vi "Teleop Drivetrain Control.vi"(10 "Button Cluster":T1, 11 "Axes":T2) -> ()   [LabVIEW 2015]
uses:
  Common Code/Gamepads/Axes Cluster.ctl
  Common Code/Gamepads/Button Cluster.ctl
  Common Code/Drivetrain Modes.ctl
  Common Code/Shot Type.ctl
  Common Code/Change Detect.vi
  Common Code/Change Detect Boolean.vi
  Robot Global Data.vi
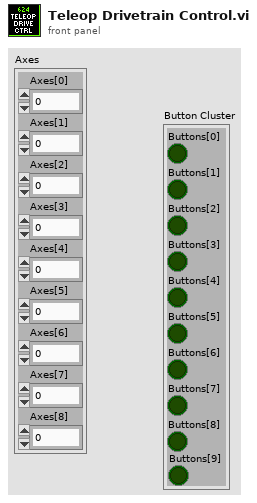
[diagram p1: front panel]
types:
  T1 = typedef "Button Cluster.ctl" = cluster{"Buttons[0]":bool, "Buttons[1]":bool, "Buttons[2]":bool, "Buttons[3]":bool, "Buttons[4]":bool, "Buttons[5]":bool, "Buttons[6]":bool, "Buttons[7]":bool, "Buttons[8]":bool, "Buttons[9]":bool}
  T2 = typedef "Axes Cluster.ctl" = cluster{"Axes[0]":dbl, "Axes[1]":dbl, "Axes[2]":dbl, "Axes[3]":dbl, "Axes[4]":dbl, "Axes[5]":dbl, "Axes[6]":dbl, "Axes[7]":dbl, "Axes[8]":dbl}
  T3 = typedef "Drivetrain Modes.ctl" = enum16{"Climb", "Manual", "Ball Vision Targeting", "Goal Vision Targeting", "PID Distance Drive", "Hybrid"}
  T4 = typedef "Shot Type.ctl" = enum16{"Batter Shot", "Corner Shot", "Curve Shot", "Vision Shot", "Deep Middle Shot"}
  T5 = typedef "Climb Command Cluster.ctl" = cluster{"Climb Mode":T6, "Hold?":bool, "Manual State":T7}
  T6 = typedef "Climb Mode.ctl" = enum16{"Auto", "Manual"}
  T7 = typedef "Climb Manual State.ctl" = cluster{"Release":bool, " PTO Engage":bool}
  T8 = typedef "Drivetrain Commands.ctl" = cluster{"Y Power":dbl, "Turn Power":dbl, "1st Gear?":bool, "Modes":T3, "Heading Target":dbl, "X Max Speed":dbl, "Y Max Speed":dbl, "X Min Speed":dbl, "Y Min Speed":dbl, "Y Target":dbl, "Max Accel":dbl, "Max Velocity":dbl}
  T9 = typedef "Shooter Command Cluster.ctl" = cluster{"Command":T10, "Mode":T11, "Shot Type":T4, "Override Trigger IR":bool}
  T10 = typedef "Shooter Commands.ctl" = enum16{"Idle", "Prime Shooter", "Shoot"}
  T11 = typedef "Shoot Modes Enum.ctl" = enum16{"Manual", "Safe", "Auto"}
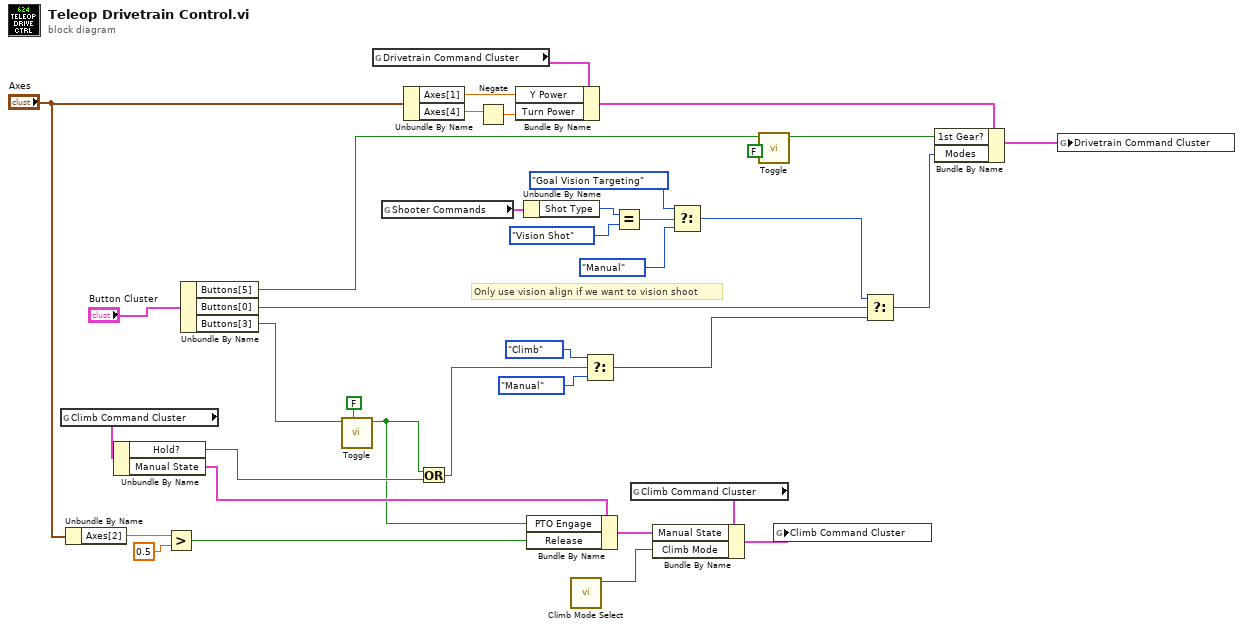
[diagram p0: block diagram]
diagram:
  # "Only use vision align if we want to vision shoot"
  n1 = global read "Robot Global Data.vi" "Climb Command Cluster"() -> (w17:T5)
  n2 = Unbundle By Name("Axes") -> ("Axes[2]"=w8:dbl)
  n3 = Unbundle By Name(w17) -> ("Hold?"=w16:bool, "Manual State"=w14:T7)
  n4 = Greater?(x=w8, y=0.5) -> (0:w6:bool)
  n5 = Unbundle By Name("Button Cluster") -> ("Buttons[5]"=w36:bool, "Buttons[0]"=w30:bool, "Buttons[3]"=w11:bool)
  n6 = call "Toggle.vi"("Initial Value"=FALSE, "In"=w11) -> ("Toggled"=w13:bool)  [unwired: 9 in]
  n7 = global read "Robot Global Data.vi" "Drivetrain Command Cluster"() -> (w31:T8)
  n8 = global read "Robot Global Data.vi" "Shooter Commands"() -> (w28:T9)
  n9 = Unbundle By Name("Axes") -> ("Axes[1]"=w4:dbl, "Axes[4]"=w3:dbl)
  n10 = Or(x=w13, y=w16) -> (x .or. y?=w15:bool)
  n11 = Negate(x=w3) -> (-x=w2:dbl)
  n12 = Bundle By Name(cluster=w31, "Y Power"=w4, "Turn Power"=w2) -> (w34:T8)
  n13 = Unbundle By Name(w28) -> ("Shot Type"=w27:T4)
  n14 = Bundle By Name(cluster=w14, "PTO Engage"=w13, "Release"=w6) -> (w12:T7)
  n15 = call "Climb Mode Select.vi"() -> ("Mode"=w5:T6)  [unwired: 11 in]
  n16 = Select(t=Drivetrain_Modes."Climb", s=w15, f=Drivetrain_Modes."Manual" ("Modes")) -> (s? t:f=w1:T3)
  n17 = Equal?(x=w27, y=Shot_Type."Vision Shot") -> (x = y?=w25:bool)
  n18 = global read "Robot Global Data.vi" "Climb Command Cluster"() -> (w18:T5)
  n19 = Bundle By Name(cluster=w18, "Manual State"=w12, "Climb Mode"=w5) -> (w10:T5)
  n20 = Select(t=Drivetrain_Modes."Goal Vision Targeting" ("Modes"), s=w25, f=Drivetrain_Modes."Manual") -> (s? t:f=w22:T3)
  n21 = call "Toggle.vi"("Initial Value"=FALSE, "In"=w36) -> ("Toggled"=w33:bool)  [unwired: 9 in]
  n22 = global write "Robot Global Data.vi" "Climb Command Cluster"(w10) -> ()
  n23 = Select(t=w22, s=w30, f=w1) -> (s? t:f=w29:T3)
  n24 = Bundle By Name(cluster=w34, "1st Gear?"=w33, "Modes"=w29) -> (w32:T8)
  n25 = global write "Robot Global Data.vi" "Drivetrain Command Cluster"(w32) -> ()
